vi "Set Delay Method (Fixed).vi"(8 "error in (no error)":errorcluster, 10 "Absolute Delay (ps)":i32=10 min=10 max=150 step=1, 11 "Abstract Delay Line in":refnum<class "Abstract Delay Line.lvclass">) -> (0 "error out":errorcluster, 3 "Abstract Delay Line out":refnum<class "Abstract Delay Line.lvclass">)   [LabVIEW 2016, in "Delay Line.lvlib" / "Abstract Delay Line.lvclass"]
uses:
  Abstract Delay Line.lvclass
  Typedef/Delay Method.ctl
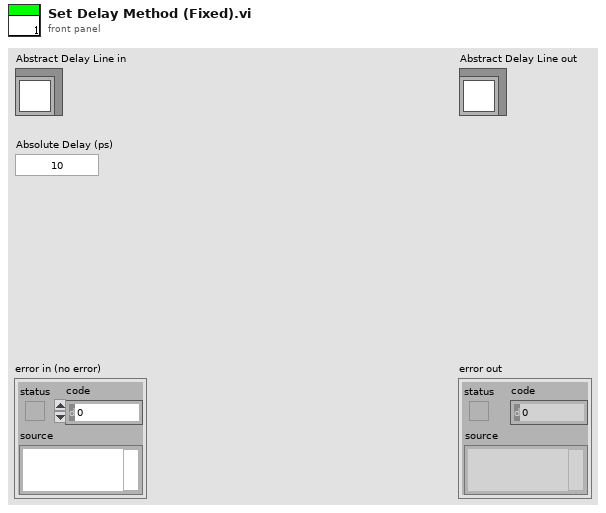
[diagram p1: front panel]
types:
  T1 = typedef "Delay Line.lvlib/Abstract Delay Line.lvclass/Delay Method.ctl" = enum8{"Periodic", "Fixed"}
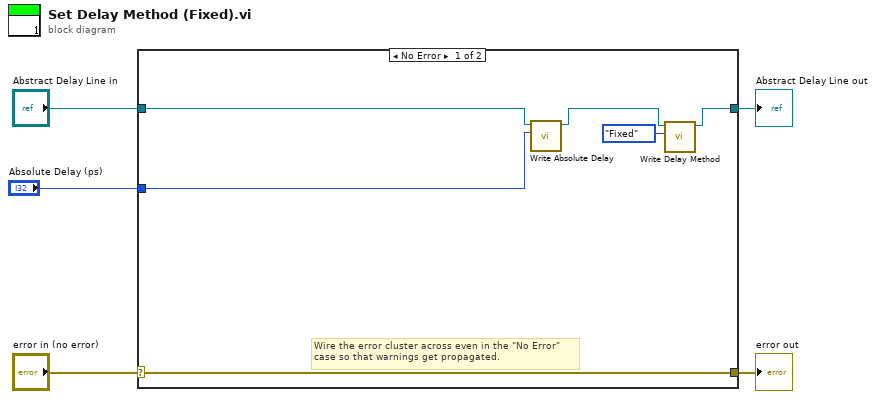
[diagram p0: block diagram]
diagram:
  n1 = case shown="No Error" "error in (no error)" {
    selector: "error in (no error)" -> [w11 w13]
    tunnel: [w11 w13] -> w4
    tunnel: [w7 w12] -> w2
    tunnel: "Abstract Delay Line in" -> [w10 w12]
    tunnel: "Absolute Delay (ps)" -> [w9 _]
    frame No Error {
      # "Wire the error cluster across even in the \"No Error\"\ncase so that warnings get propagated."
      n2 = call-dynamic "Write Absolute Delay.vi"("Absolute Delay (ps)"=w9, "Abstract Delay Line in"=w10) -> ("Abstract Delay Line out"=w8:refnum<class "Abstract Delay Line.lvclass">)  [unwired: 9 in]
      n3 = call-dynamic "Write Delay Method.vi"("Delay Method"=Delay_Method."Fixed", "Abstract Delay Line in"=w8) -> ("Abstract Delay Line out"=w7:refnum<class "Abstract Delay Line.lvclass">)  [unwired: 9 in]
    }
    frame Error {
    }
  }
  "error out" <- w4
  "Abstract Delay Line out" <- w2
